vi "Display Image.vi"(11 "Data":T1={"Frame ID"=832, "Data"=array[4147200 elements]}) -> ()   [LabVIEW 2026]
uses:
  ttashjia/GSE/Host/Common/Types/Serial Channel Display Parameters.ctl
  <vilib>/vision/Image Controls.llb/IMAQ Image.ctl
  ttashjia/GSE/Host/Common/Types/RAW Interpretation for Display.ctl
  ttashjia/GSE/FPGA/Common/Types/Image Metadata.ctl
  <instrlib>/FlexRIO/CSI-2/v2/Common/Types/LLP Data Type.ctl
  image.ctl
  ttashjia/GSE/Host/Common/GettingStarted_Common_148X_Host.lvlib
  <instrlib>/FlexRIO/CSI-2/v2/Common/NI CSI-2 API Common v2.lvlib
  ttashjia/GSE/FPGA/Common/GettingStarted_Common_148X_FPGA.lvlib
  Automotive Vision.lvclass
panel:
  out "size(s)":i32=4147200
  in  "stop":bool
  out "1st channel display":T2(plugin-control)
  in  "error in (no error)":errorcluster
  in  "display channel number":i32
  out "error out":errorcluster
  in  "image metadata":T3={"serial channel"=0.0, "frame number"=0, "data type"=enum."RAW 12", "width"=1920, "height"=1080, "image bytes"=0, "total bytes"=0, "little endian"=FALSE}
  in  "serial channel display parameters":T5[](array[typedef])=[{"images"={"grayscale"=refnum, "color"=refnum}, "RAW parameters"={"interpretation"=enum."Grayscale", "bayer parameters"={"pattern"=0, "algorithm"=0, "red gain"=0.0, "green gain"=0.0, "blue gain"=0.0}}}] {"RAW parameters"."bayer parameters"."blue gain" format="%_4g"; "RAW parameters"."bayer parameters"."green gain" format="%_4g"; "RAW parameters"."bayer parameters"."red gain" format="%_4g"; "RAW parameters"."bayer parameters"."algorithm" items=["Bilinear", "VNG"]; "RAW parameters"."bayer parameters"."pattern" items=["GB", "GR", "BG", "RG"]}
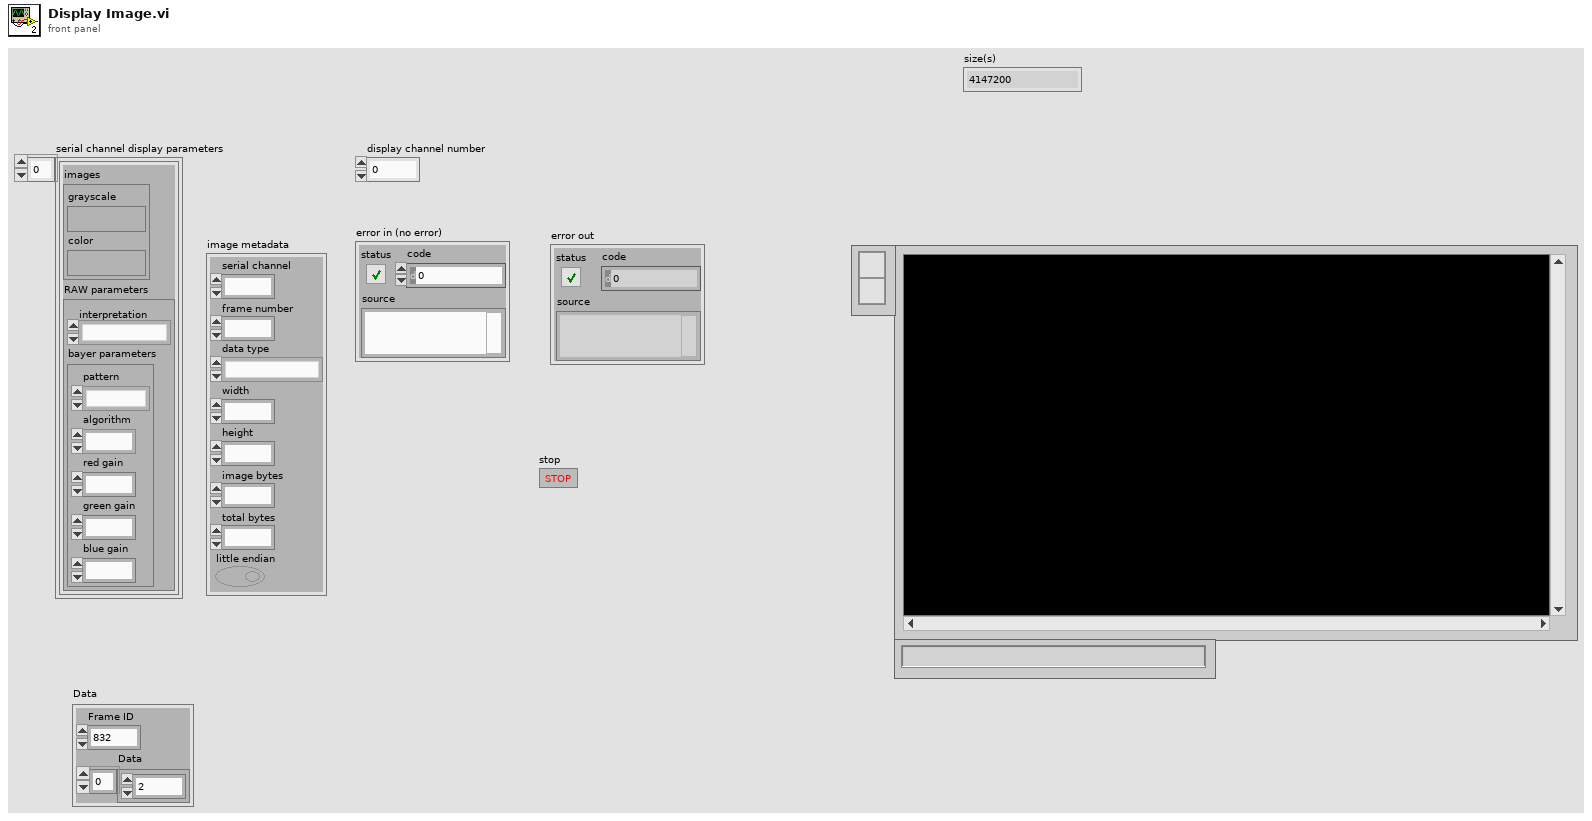
[diagram p1: front panel]
types:
  T1 = typedef "Automotive Vision.lvclass/image.ctl" = cluster{"Frame ID":u32, "Data":u8[]}
  T2 = typedef "IMAQ Image.ctl" = refnum<image>
  T3 = typedef "GettingStarted_Common_148X_FPGA.lvlib/Image Metadata.ctl" = cluster{"serial channel":fxp<+,3,3>, "frame number":u16, "data type":T4, "width":u16, "height":u16, "image bytes":u32, "total bytes":u32, "little endian":bool}
  T4 = typedef "NI CSI-2 API Common v2.lvlib/LLP Data Type.ctl" = enum8{"Frame Start", "Frame End", "Line Start", "Line End", "End of Transmission", "Reserved 0", "Reserved 1", "Reserved 2", "Generic Short Packet 1", "Generic Short Packet 2", "Generic Short Packet 3", "Generic Short Packet 4", "Generic Short Packet 5", "Generic Short Packet 6", "Generic Short Packet 7", "Generic Short Packet 8", "Null", "Blanking Data", "Embedded 8-bit non Image Data", "Generic Long Packet 1", "Generic Long Packet 2", "Generic Long Packet 3", "Generic Long Packet 4", "Reserved 3", "YUV420 8-bit", "YUV420 10-bit", "Legacy YUV420 8-bit", "Reserved 4", "YUV420 8-bit Chroma Shifted", "YUV420 10-bit Chroma Shifted", "YUV422 8-bit", "YUV422 10-bit", "RGB444", "RGB555", "RGB565", "RGB666", "RGB888", "Reserved 5", "Reserved 6", "RAW 24", "RAW 6", "RAW 7", "RAW 8", "RAW 10", "RAW 12", "RAW 14", "RAW 16", "RAW 20", "User Defined 8-bit Data 1", "User Defined 8-bit Data 2", "User Defined 8-bit Data 3", "User Defined 8-bit Data 4", "User Defined 8-bit Data 5", "User Defined 8-bit Data 6", "User Defined 8-bit Data 7", "User Defined 8-bit Data 8", "USL Command", "Reserved 7", "Reserved 8", "Reserved 9", "Reserved 10", "Reserved 11", "Reserved 12", "LRTE EPD Spacer"}
  T5 = typedef "GettingStarted_Common_148X_Host.lvlib/Serial Channel Display Parameters.ctl" = cluster{"images":cluster{"grayscale":T2, "color":T2}, "RAW parameters":cluster{"interpretation":T6, "bayer parameters":cluster{"pattern":i32, "algorithm":i32, "red gain":dbl, "green gain":dbl, "blue gain":dbl}}}
  T6 = typedef "GettingStarted_Common_148X_Host.lvlib/RAW Interpretation for Display.ctl" = enum16{"Grayscale", "Bayer", "RGB", "YUV422", "YUV420", "Legacy YUV420"}
  T7 = typedef "Image Type" = u32
  T8 = cluster{"pattern":i32, "algorithm":i32, "red gain":dbl, "green gain":dbl, "blue gain":dbl}
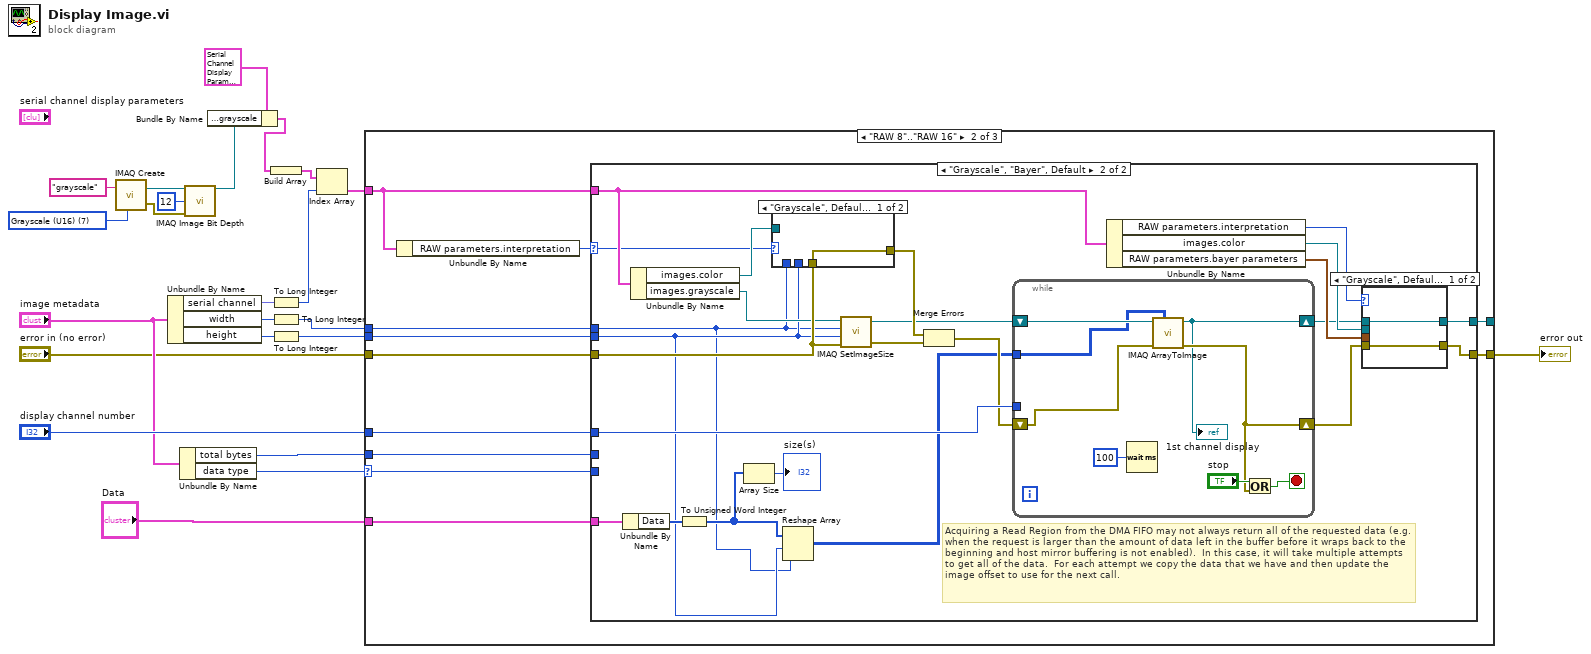
[diagram p0: block diagram]
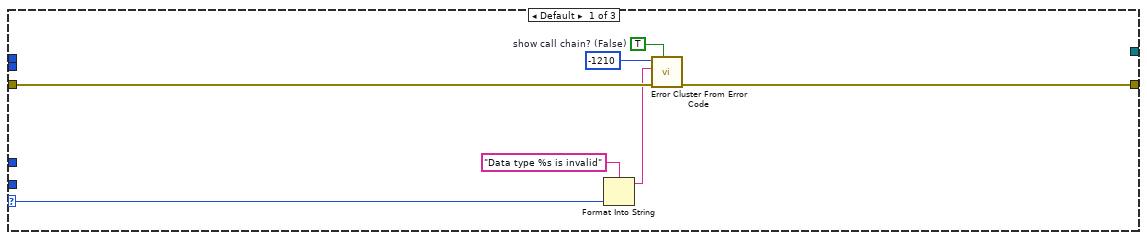
[diagram p2: hidden frame]
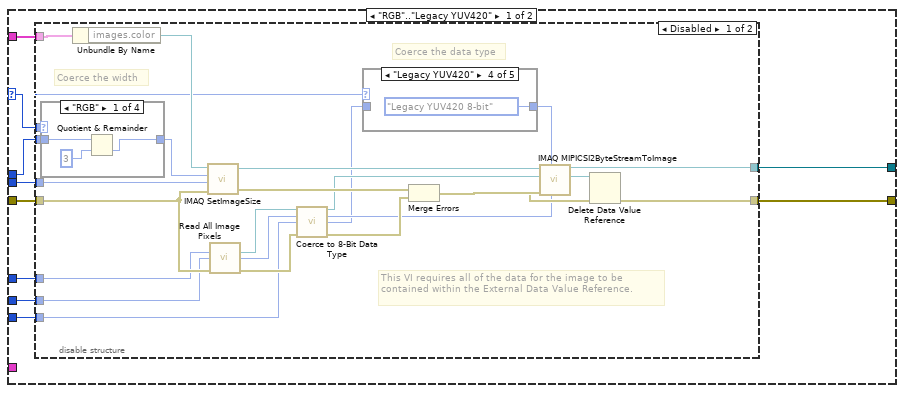
[diagram p3: hidden frame]
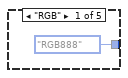
[diagram p4: hidden frame]
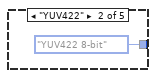
[diagram p5: hidden frame]
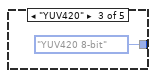
[diagram p6: hidden frame]
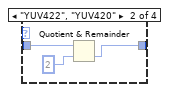
[diagram p8: hidden frame]
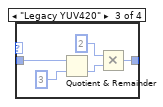
[diagram p9: hidden frame]
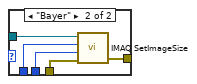
[diagram p12: hidden frame]
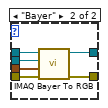
[diagram p13: hidden frame]
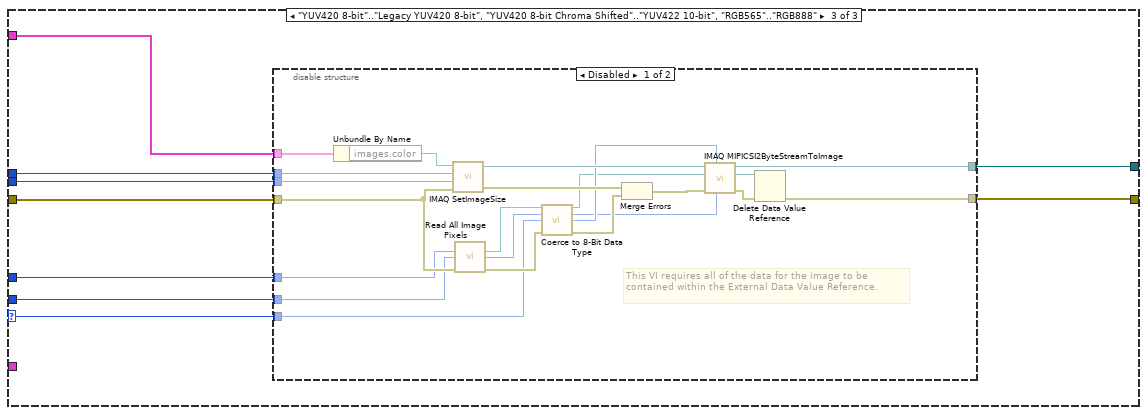
[diagram p14: hidden frame]
diagram:
  w4 = T7 7 items=["Grayscale (U8)", "Grayscale (I16)", "Grayscale (SGL)", "Complex (CSG)", "RGB (U32)", "HSL (U32)", "RGB (U64)", "Grayscale (U16)"] ("Image Type")
  n1 = call "IMAQ Create"("Image Name"="grayscale", "Image Type"=w4) -> ("New Image"=w9:T2, "error out"=w3:errorcluster)  [unwired: 3 in]
  n2 = Unbundle By Name("image metadata") -> ("serial channel"=w21:fxp<+,3,3>, "width"=w17:u16, "height"=w18:u16)
  n3 = Unbundle By Name("image metadata") -> ("total bytes"=w23:u32, "data type"=w11:T4)
  n4 = call "IMAQ Image Bit Depth"("Image"=w9, "Bit Depth (0)"=u32 12, "error in (no error)"=w3) -> ("Image Out"=w2:T2)  [unwired: 10 in, 2 out]
  n5 = Bundle By Name(cluster=T5 {"images"={"grayscale"=refnum, "color"=refnum}, "RAW parameters"={"interpretation"=enum."Grayscale", "bayer parameters"={"pattern"=0, "algorithm"=0, "red gain"=0.0, "green gain"=0.0, "blue gain"=0.0}}} ("pixels to image params"), "images.grayscale"=w2) -> (w1:T5)
  n6 = Build Array(w1) -> (w5:T5[])
  n7 = To Long Integer(number=w21) -> (32bit integer=w19:i32)
  n8 = To Long Integer(number=w17) -> (32bit integer=w14:i32)
  n9 = To Long Integer(number=w18) -> (32bit integer=w15:i32)
  n10 = Index Array(array=w5, index=w19) -> (element=w12:T5)
  n11 = case shown="\"RAW 8\"..\"RAW 16\"" w11 {
    selector: w11 -> [w24 w32 w141]
    tunnel: w23 -> [_ w41 w145]
    tunnel: "display channel number" -> [_ w40 w144]
    tunnel: "error in (no error)" -> [w28 w39 w146]
    tunnel: w15 -> [_ w38 w149]
    tunnel: w14 -> [_ w37 w148]
    tunnel: [_ w36 w143] -> _
    tunnel: [w27 w35 w142] -> w13
    tunnel: w12 -> [_ w34 w147]
    tunnel: "Data" -> [_ w31 _]
    frame Default {
      w29 = TRUE  # show call chain? (False)
      n12 = Format Into String(format string="Data type %s is invalid" ("error message (\"\")"), w24) -> (resulting string=w25:string)  [unwired: 2 in, 1 out]
      n13 = call <vilib>:"Error Cluster From Error Code.vi"("show call chain? (False)"=w29, "error in (no error)"=w28, "error message (\"\")"=w25, "error code (0)"=-1210) -> ("error out"=w27:errorcluster)  [unwired: 5 in]
    }
    frame "RAW 8".."RAW 16" {
      n14 = Unbundle By Name(w34) -> ("RAW parameters.interpretation"=w33:T6)
      n15 = case shown="\"Grayscale\", \"Bayer\", Default" w33 {
        selector: w33 -> [w42 w104]
        tunnel: w41 -> [w48 _]
        tunnel: w40 -> [w47 w117]
        tunnel: w39 -> [w51 w116]
        tunnel: w38 -> [w44 w96]
        tunnel: w37 -> [w43 w95]
        tunnel: [w49 w113] -> w36
        tunnel: [w50 w111] -> w35
        tunnel: w34 -> [w46 w107]
        tunnel: w32 -> [w45 _]
        tunnel: w31 -> [_ w103]
        frame "RGB".."Legacy YUV420" {
          n16 = disable-structure shown="Disabled" {
            disable-tunnel: w51 -> [w64 w94]
            disable-tunnel: [w63 w94] -> w50
            disable-tunnel: [w62 _] -> w49
            disable-tunnel: w48 -> [w61 _]
            disable-tunnel: w47 -> [w60 _]
            disable-tunnel: w46 -> [w59 _]
            disable-tunnel: w45 -> [w58 _]
            disable-tunnel: w44 -> [w57 _]
            disable-tunnel: w43 -> [w56 _]
            disable-tunnel: w42 -> [w54 _]
            frame Disabled {
              # "Coerce the data type"
              # "Coerce the width"
              # "This VI requires all of the data for the image to be contained within the External Data Value Reference."
              n17 = case shown="\"RGB\"" w54 {
                tunnel: w56 -> [w83 w86 w92 w93]
                tunnel: [w82 w85 w89 w93] -> w55
                frame "RGB" {
                  n18 = Quotient & Remainder(x=w83, y=3) -> (floor(x/y)=w82:i32)  [unwired: 1 out]
                }
                frame "YUV422", "YUV420" {
                  n19 = Quotient & Remainder(x=w86, y=2) -> (floor(x/y)=w85:i32)  [unwired: 1 out]
                }
                frame "Legacy YUV420" {
                  n20 = Quotient & Remainder(x=w92, y=3) -> (floor(x/y)=w90:i32)  [unwired: 1 out]
                  n21 = Multiply(x=2, y=w90) -> (x*y=w89:i32)
                }
                frame Default {
                }
              }
              n22 = Unbundle By Name(w59) -> ("images.color"=w76:T2)
              n23 = call "IMAQ SetImageSize"("error in (no error)"=w64, "Y Resolution"=w57, "X Resolution"=w55, "Image"=w76) -> ("error out"=w74:errorcluster, "Image Out"=w75:T2)  [unwired: 1 in]
              n24 = call "Read All Image Pixels.vi"("display channel number"=w60, "image bytes"=w61, "error in (no error)"=w64) -> ("image pixel data region"=w69:refnum<data-value>, "elements in region"=w68:u32, "error out"=w70:errorcluster)  [unwired: 9 in, 1 out]
              n25 = call "Coerce to 8-Bit Data Type.vi"("image pixel data region in"=w69, "image bytes in"=w68, "data type in"=w58, "error in (no error)"=w70) -> ("image pixel data region out"=w65:refnum<data-value>, "image bytes out"=w66:u32, "data type out"=w52:T4, "error out"=w67:errorcluster)  [unwired: 8 in]
              n26 = case shown="\"Legacy YUV420\"" w54 {
                tunnel: w52 -> [_ _ _ _ w81]
                tunnel: [LLP_Data_Type."RGB888" ("data type") LLP_Data_Type."YUV422 8-bit" ("data type") LLP_Data_Type."YUV420 8-bit" ("data type") LLP_Data_Type."Legacy YUV420 8-bit" ("data type") w81] -> w53
                frame "RGB" {
                }
                frame "YUV422" {
                }
                frame "YUV420" {
                }
                frame "Legacy YUV420" {
                }
                frame Default {
                }
              }
              n27 = Merge Errors(w74, w67) -> (w73:errorcluster)
              n28 = call "IMAQ MIPICSI2ByteStreamToImage"("Bytes to Copy"=w66, "Format"=w53, "error in (no error)"=w73, "Byte Stream In"=w65, "Image In"=w75) -> ("error out"=w72:errorcluster, "Byte Stream Out"=w71:refnum<data-value>, "Image Out"=w62:T2)  [unwired: 3 in, 1 out]
              n29 = Delete Data Value Reference(data value reference=w71, error in=w72) -> (error out=w63:errorcluster)  [unwired: 1 out]
            }
            frame Enabled {
            }
          }
        }
        frame "Grayscale", "Bayer", Default {
          # "Acquiring a Read Region from the DMA FIFO may not always return all of the requested data (e.g. when the request is larger than the amount of data left in the buffer before it wraps back to the beginning and host mirror buffering is not enabled).  In this case, it will take multiple attempts to get all of the data.  For each attempt we copy the data that we have and then update the image offset to use for the next call."
          n30 = Unbundle By Name(w103) -> ("Data"=w101:u8[])
          n31 = Unbundle By Name(w107) -> ("images.color"=w114:T2, "images.grayscale"=w99:T2)
          n32 = To Unsigned Word Integer(number=w101) -> (unsigned 16bit integer=w98:u16[])
          n33 = Array Size(array=w98) -> (size(s)=→"size(s)":i32)
          n34 = case shown="\"Grayscale\", Default" w104 {
            tunnel: w116 -> [w119 w124]
            tunnel: [w119 w123] -> w115
            tunnel: w114 -> [_ w122]
            tunnel: w96 -> [_ w121]
            tunnel: w95 -> [_ w120]
            frame "Grayscale", Default {
            }
            frame "Bayer" {
              n35 = call "IMAQ SetImageSize"("error in (no error)"=w124, "Y Resolution"=w121, "X Resolution"=w120, "Image"=w122) -> ("error out"=w123:errorcluster)  [unwired: 1 in, 1 out]
            }
          }
          n36 = Reshape Array(w98, w96, w95) -> (w102:u16[][])
          n37 = call "IMAQ SetImageSize"("error in (no error)"=w116, "Y Resolution"=w96, "X Resolution"=w95, "Image"=w99) -> ("error out"=w118:errorcluster, "Image Out"=w106:T2)  [unwired: 1 in]
          n38 = Merge Errors(w115, w118) -> (w105:errorcluster)
          n39 = while {
            tunnel: w117 -> [_]
            shift-right: [w127] -> w112
            shift-left: w105 -> [w132]
            tunnel: w102 -> [w126]
            shift-right: [w125] -> w97
            shift-left: w106 -> [w131]
            stop <- w128 stop-if-true
            n40 = Wait (ms)(milliseconds to wait=u32 100) -> ()  [unwired: 1 out]
            n41 = call "IMAQ ArrayToImage"("Image Pixels (U16)"=w126, "error in (no error)"=w132, "Image"=w131) -> ("error out"=w127:errorcluster, "Image Out"=w125:T2)  [unwired: 7 in]
            "1st channel display" <- w125
            n42 = Or(x="stop", y=w127) -> (x .or. y?=w128:bool)
          }
          n43 = Unbundle By Name(w107) -> ("RAW parameters.interpretation"=w108:T6, "images.color"=w109:T2, "RAW parameters.bayer parameters"=w110:T8)
          n44 = case shown="\"Grayscale\", Default" w108 {
            tunnel: w97 -> [w133 w140]
            tunnel: [w133 w139] -> w113
            tunnel: w112 -> [w134 w138]
            tunnel: [w134 w137] -> w111
            tunnel: w109 -> [_ w136]
            tunnel: w110 -> [_ w135]
            frame "Grayscale", Default {
            }
            frame "Bayer" {
              n45 = call "IMAQ Bayer To RGB"("error in (no error)"=w138, "Bayer Parameters"=w135, "Image Dst"=w136, "Image Src"=w140) -> ("error out"=w137:errorcluster, "Image Dst Out"=w139:T2)  [unwired: 6 in]
            }
          }
        }
      }
    }
    frame "YUV420 8-bit".."Legacy YUV420 8-bit", "YUV420 8-bit Chroma Shifted".."YUV422 10-bit", "RGB565".."RGB888" {
      n46 = disable-structure shown="Disabled" {
        disable-tunnel: w149 -> [w171 _]
        disable-tunnel: w148 -> [w170 _]
        disable-tunnel: w147 -> [w168 _]
        disable-tunnel: w146 -> [w165 w172]
        disable-tunnel: w145 -> [w163 _]
        disable-tunnel: w144 -> [w162 _]
        disable-tunnel: [w161 _] -> w143
        disable-tunnel: [w158 w172] -> w142
        disable-tunnel: w141 -> [w153 _]
        frame Disabled {
          # "This VI requires all of the data for the image to be contained within the External Data Value Reference."
          n47 = Unbundle By Name(w168) -> ("images.color"=w169:T2)
          n48 = call "IMAQ SetImageSize"("error in (no error)"=w165, "Y Resolution"=w171, "X Resolution"=w170, "Image"=w169) -> ("error out"=w166:errorcluster, "Image Out"=w167:T2)  [unwired: 1 in]
          n49 = call "Read All Image Pixels.vi"("display channel number"=w162, "image bytes"=w163, "error in (no error)"=w165) -> ("image pixel data region"=w156:refnum<data-value>, "elements in region"=w155:u32, "error out"=w157:errorcluster)  [unwired: 9 in, 1 out]
          n50 = call "Coerce to 8-Bit Data Type.vi"("image pixel data region in"=w156, "image bytes in"=w155, "data type in"=w153, "error in (no error)"=w157) -> ("image pixel data region out"=w150:refnum<data-value>, "image bytes out"=w151:u32, "data type out"=w152:T4, "error out"=w154:errorcluster)  [unwired: 8 in]
          n51 = Merge Errors(w166, w154) -> (w164:errorcluster)
          n52 = call "IMAQ MIPICSI2ByteStreamToImage"("Bytes to Copy"=w151, "Format"=w152, "error in (no error)"=w164, "Byte Stream In"=w150, "Image In"=w167) -> ("error out"=w160:errorcluster, "Byte Stream Out"=w159:refnum<data-value>, "Image Out"=w161:T2)  [unwired: 3 in, 1 out]
          n53 = Delete Data Value Reference(data value reference=w159, error in=w160) -> (error out=w158:errorcluster)  [unwired: 1 out]
        }
        frame Enabled {
        }
      }
    }
  }
  "error out" <- w13
